vi "Chroma 1905x Series Source Settings in Step.vi"(8 "error in (no error)":errorcluster, 11 "VISA resource name":refnum<visa-resource-name>) -> (0 "error out":errorcluster, 2 "Settings":string, 3 "VISA resource name out":refnum<visa-resource-name>)   [LabVIEW 2025]
doc: "Chroma\n5 Clock Tower Place Suite 210\nMaynard, MA 01754\nTel: 1 800 253-1230\nTel: 1 877 4 A HIPOT\nFax: 1 978-461-4295\nWebsite: www.chroma.com"
uses:
  <instrlib>/Chroma 19052/Chroma 19052.lvlib
panel:
  in  "Step":u32=1 min=1 max=99 step=1
  # "Settings by Step"
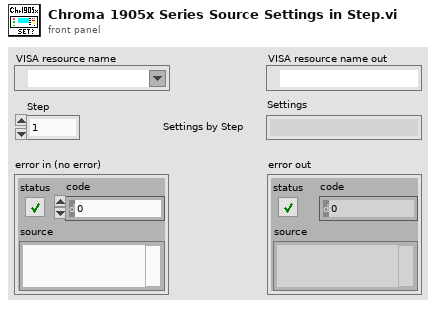
[diagram p1: front panel]
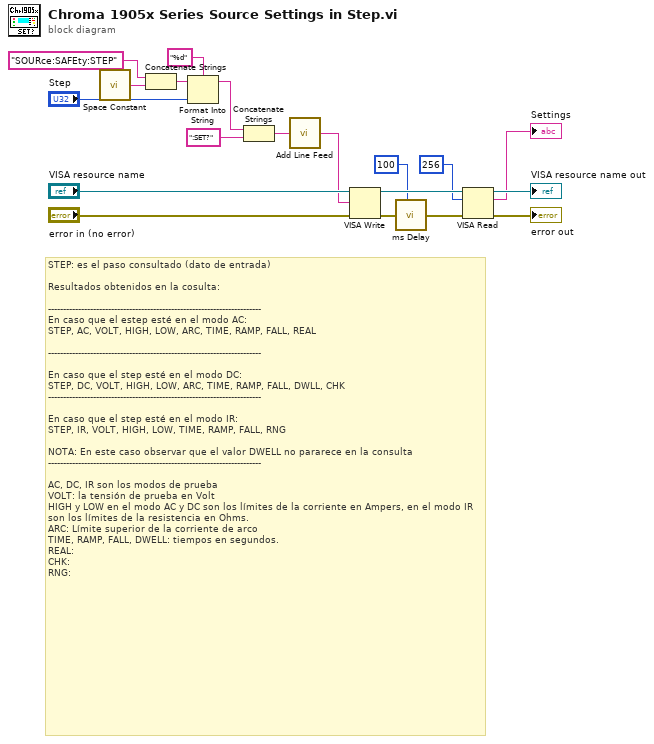
[diagram p0: block diagram]
diagram:
  # "STEP: es el paso consultado (dato de entrada)\n\nResultados obtenidos en la cosulta:\n\n-----------------------------------------------------------------------\nEn caso que el estep esté en el modo AC:\nSTEP, AC, VOLT, HIGH, LOW, ARC, TIME, RAMP, FALL, REAL\n\n-----------------------------------------------------------------------\n\nEn caso que el step esté en el modo DC:\nSTEP, DC, VOLT, HIGH, LOW, ARC, TIME, RAMP, FALL, DWLL, CHK\n-----------------------------------------------------------------------\n\nEn caso que el step esté en el modo IR:\nSTEP, IR, VOLT, HIGH, LOW, TIME, RAMP, FALL, RNG\n\nNOTA: En este caso observar que el valor DWELL no pararece en la consulta\n-----------------------------------------------------------------------\n\nAC, DC, IR son los modos de prueba\nVOLT: la tensión de prueba en Volt\nHIGH y LOW en el modo AC y DC son los límites de la corriente en Ampers, en el modo IR son los límites de la resistencia en Ohms.\nARC: Límite superior de la corriente de arco\nTIME, RAMP, FALL, DWELL: tiempos en segundos.\nREAL: \nCHK:\nRNG:"
  n1 = call <vilib>:"Space Constant.vi"() -> ("String"=w5:string)
  n2 = Concatenate Strings("SOURce:SAFEty:STEP", w5) -> (w4:string)
  n3 = Format Into String(format string="%d", initial string=w4, "Step") -> (resulting string=w9:string)  [unwired: 1 in, 1 out]
  n4 = Concatenate Strings(w9, ":SET?") -> (w7:string)
  n5 = call <instrlib>:"Add Line Feed.vi"("Command string"=w7) -> ("Concatenated string"=w15:string)  [unwired: 4 in]
  n6 = VISA Write(VISA resource name="VISA resource name", write buffer=w15, error in (no error)="error in (no error)") -> (VISA resource name out=w19:refnum<visa-resource-name>, error out=w3:errorcluster)  [unwired: 1 out]
  n7 = call <instrlib>:"ms Delay.vi"("miliseconds to wait"=u32 100 ("Time Delay ms"), "error in (no error)"=w3) -> ("error out"=w2:errorcluster)  [unwired: 6 in, 1 out]
  n8 = VISA Read(VISA resource name=w19, byte count=u32 256, error in (no error)=w2) -> (VISA resource name out=→"VISA resource name out":refnum<visa-resource-name>, read buffer=→"Settings":string, error out=→"error out":errorcluster)  [unwired: 1 out]
